vi "Configure Digital Gen IMDSig.vi"(0 "VISA resource name":refnum<visa-resource-name>, 1 "IM Frequency (10 Hz)":dbl=10.0, 2 "Waveform Type (0: imdSMPTE)":i32(ring) items=["imdSMPTE", "imdCCIF", "imdDIMB", "imdDIM30", "imdDIM100"], 5 "Channel (0: chA)":i32(ring) items=["chA", "chB"], 7 "Amplitude (0 FFS)":dbl, 9 "Amplitude Ratio (0: ar41)":i32(ring) items=["ar41", "ar11"], 11 "error in (no error)":errorcluster, 12 "Main Frequency (50 Hz)":dbl=50.0, 13 "Enable Waveform (T: Enable)":bool=TRUE) -> (4 "VISA resource name out":refnum<visa-resource-name>, 15 "error out":errorcluster)   [LabVIEW 2014, in "Stanford Research SR1.lvlib"]
doc: "Configures the attributes for the Digital Generator IMDSig."
uses:
  Stanford Research SR1.lvlib
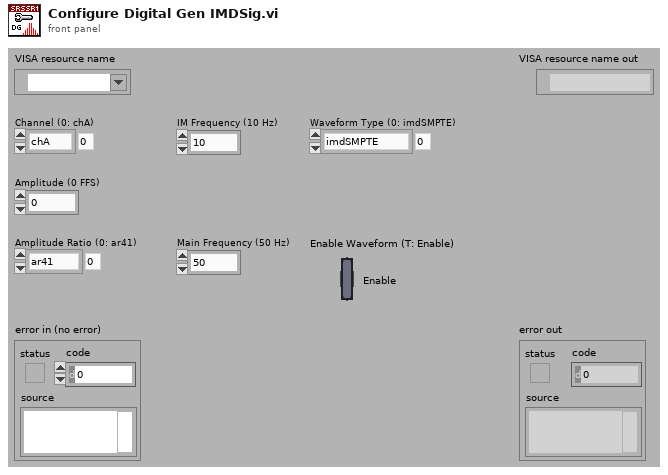
[diagram p1: front panel]
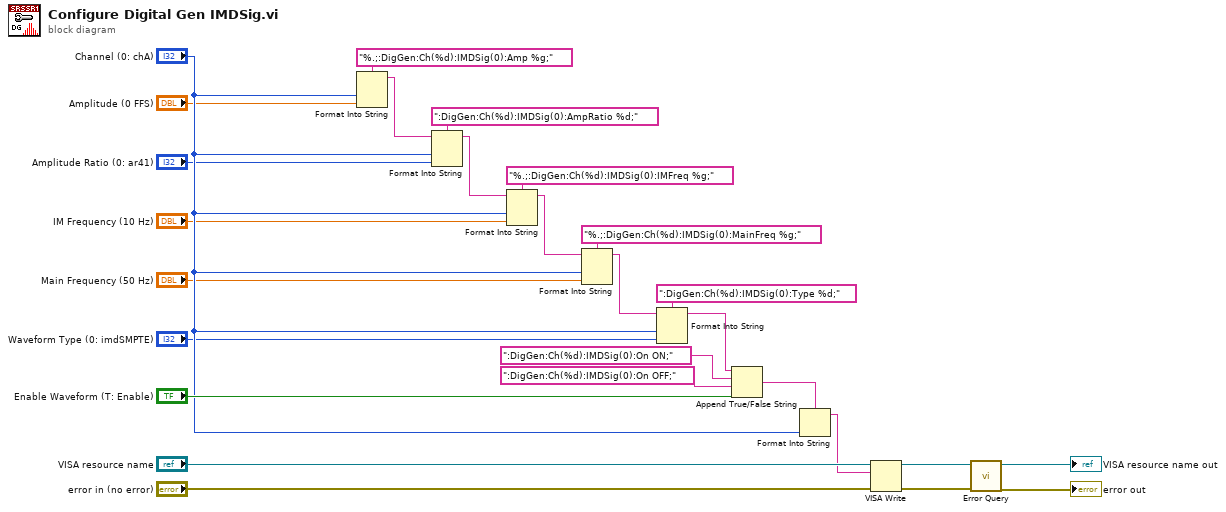
[diagram p0: block diagram]
diagram:
  n1 = Format Into String(format string="%.;:DigGen:Ch(%d):IMDSig(0):Amp %g;", "Channel (0: chA)", "Amplitude (0 FFS)") -> (resulting string=w26:string)  [unwired: 2 in, 1 out]
  n2 = Format Into String(format string=":DigGen:Ch(%d):IMDSig(0):AmpRatio %d;", initial string=w26, "Channel (0: chA)", "Amplitude Ratio (0: ar41)") -> (resulting string=w24:string)  [unwired: 1 in, 1 out]
  n3 = Format Into String(format string="%.;:DigGen:Ch(%d):IMDSig(0):IMFreq %g;", initial string=w24, "Channel (0: chA)", "IM Frequency (10 Hz)") -> (resulting string=w22:string)  [unwired: 1 in, 1 out]
  n4 = Format Into String(format string="%.;:DigGen:Ch(%d):IMDSig(0):MainFreq %g;", initial string=w22, "Channel (0: chA)", "Main Frequency (50 Hz)") -> (resulting string=w20:string)  [unwired: 1 in, 1 out]
  n5 = Format Into String(format string=":DigGen:Ch(%d):IMDSig(0):Type %d;", initial string=w20, "Channel (0: chA)", "Waveform Type (0: imdSMPTE)") -> (resulting string=w18:string)  [unwired: 1 in, 1 out]
  n6 = Append True/False String(1:"Enable Waveform (T: Enable)", 2:":DigGen:Ch(%d):IMDSig(0):On OFF;", 3:":DigGen:Ch(%d):IMDSig(0):On ON;", 4:w18) -> (0:w8:string)
  n7 = Format Into String(format string=w8, "Channel (0: chA)") -> (resulting string=w7:string)  [unwired: 2 in, 1 out]
  n8 = VISA Write(VISA resource name="VISA resource name", write buffer=w7, error in (no error)="error in (no error)") -> (VISA resource name out=w12:refnum<visa-resource-name>, error out=w11:errorcluster)  [unwired: 1 out]
  n9 = call "Error Query.vi"("error in (no error)"=w11, "VISA resource name"=w12) -> ("error out"=→"error out":errorcluster, "VISA resource name out"=→"VISA resource name out":refnum<visa-resource-name>)  [unwired: 6 in, 2 out]
